vi "P3060_写入U8数据.vi"(8 "错误输入":errorcluster caption="错误输入（无错误）", 9 "U8数据":u8, 10 "偏移地址":u32, 11 "句柄输入":i32) -> (0 "错误输出":errorcluster, 2 "返回值":i32, 3 "句柄输出":i32)   [LabVIEW 2010]
uses:
  dll/P3060.dll
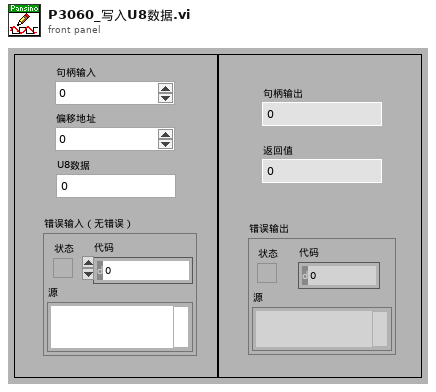
[diagram p1: front panel]
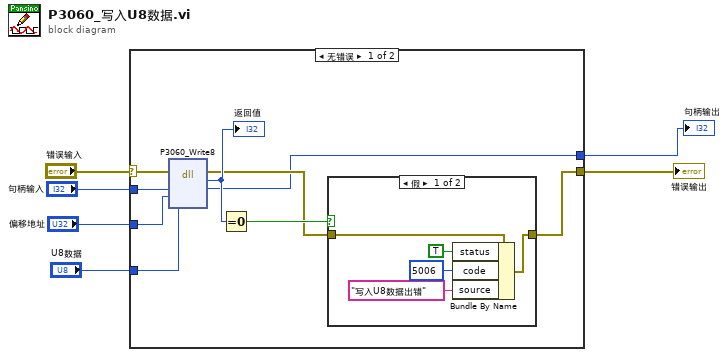
[diagram p0: block diagram]
diagram:
  n1 = case shown="无错误" "错误输入" {
    selector: "错误输入" -> [w11 w23]
    tunnel: [w15 w23] -> w4
    tunnel: "句柄输入" -> [w10 w22]
    tunnel: "偏移地址" -> [w9 _]
    tunnel: [w8 w22] -> w2
    tunnel: "U8数据" -> [w7 _]
    frame No Error {
      n2 = dll-call lib="D:/driver/trunk/Drivers/P3060/P3060API/P3060APILV/Labview/P3060/_SubVI/dll/P3060.dll" fn="P3060_Write8"(error in=w11, "hDev"=w10, "Offset"=w9, "data"=w7) -> (error out=w12:errorcluster, "return"=w14:i32, "hDev"=w8:i32)  [unwired: 4 in, 1 out]
      "返回值" <- w14
      n3 = Equal To 0?(x=w14) -> (x = 0?=w13:bool)
      n4 = case shown="假" w13 {
        tunnel: [w19 w21] -> w15
        tunnel: w12 -> [w20 w21]
        frame False {
          n5 = Bundle By Name(cluster=w20, "status"=TRUE, "code"=5006, "source"="写入U8数据出错") -> (w19:errorcluster)
        }
        frame True {
        }
      }
    }
    frame Error {
    }
  }
  "错误输出" <- w4
  "句柄输出" <- w2
